vi "Camera New Frame Arrived Callback.vi"(4 "Camera_Prime95B in":refnum<class "Camera_Prime95B.lvclass">, 5 "Event Data":cluster{"sender":refnum<k24>, "e":refnum<k24>}, 6 "Control Ref":refnum<k24>, 7 "Event Common Data":T1) -> ()   [LabVIEW 2020, in "Camera_Prime95B.lvlib" / "Camera_Prime95B.lvclass"]
uses:
  Camera_Prime95B.lvclass
  D:/Daguan/Development/MMicroscopyAF/Model/Hardware Layer/Real Hardware/Camera_Prime95B/Camera_Prime95B/Dependencies/PVCamNET.dll
  Dependencies/PVCamNET.dll
  C:/Program Files/National Instruments/LabVIEW 2020/vi.lib/ActorFramework/Actor/Actor.lvclass
  <vilib>/ActorFramework/Actor/Actor.lvclass/Actor.ctl
  <vilib>/ActorFramework/Message Enqueuer/Message Enqueuer.lvclass/Message Enqueuer.ctl
  Camera_Prime95B Messages/On New Frame Arrival Msg/On New Frame Arrival Msg.lvclass/On New Frame Arrival Msg.ctl
  <vilib>/ActorFramework/Message Enqueuer/Init from Existing Queue.vi
  <vilib>/ActorFramework/Message Enqueuer/Enqueue.vi
  Camera_Prime95B Messages/On New Frame Arrival Msg/On New Frame Arrival Msg.lvclass
  C:/Program Files/National Instruments/LabVIEW 2020/vi.lib/ActorFramework/Message/Message.lvclass
  <vilib>/ActorFramework/Message Priority Queue/Priority Enqueue.vi
  <vilib>/ActorFramework/Message Enqueuer/Message Enqueuer.lvclass
  <vilib>/ActorFramework/Actor/Actor.lvclass
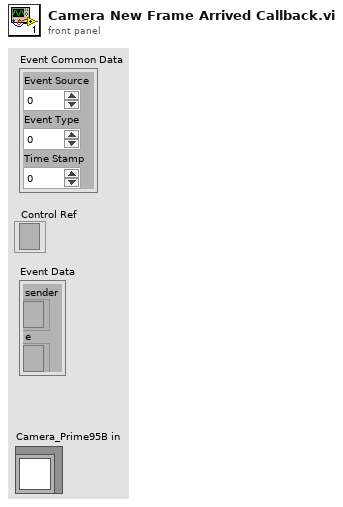
[diagram p1: front panel]
types:
  T1 = cluster{"Event Source":i32, "Event Type":u32, "Time Stamp":u32}
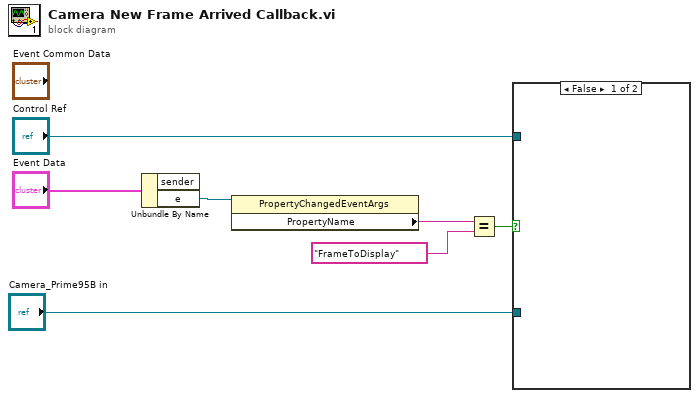
[diagram p0: block diagram]
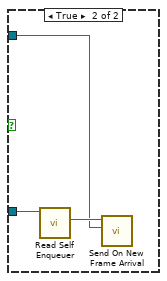
[diagram p2: hidden frame]
diagram:
  n1 = Unbundle By Name("Event Data") -> ("e"=w6:refnum<k24>)  [unwired: 1 out]
  n2 = property class="PropertyChangedEventArgs"(reference=w6) -> ("PropertyName"=w5:string)  [unwired: 1 in, 2 out]
  n3 = Equal?(x=w5, y="FrameToDisplay") -> (x = y?=w3:bool)
  n4 = case shown="False" w3 {
    tunnel: "Control Ref" -> [_ w8]
    tunnel: "Camera_Prime95B in" -> [_ w9]
    frame False {
    }
    frame True {
      n5 = call <vilib>:"Read Self Enqueuer.vi"("Actor"=w9) -> ("Self Enqueuer"=w10:refnum<class "Message Enqueuer.lvclass">)  [unwired: 10 in]
      n6 = call "Send On New Frame Arrival.vi"("Control Ref"=w8, "Message Enqueuer"=w10) -> ()  [unwired: 8 in, 2 out]
    }
  }
